vi "svfa_Check for Zoom Settings Change (1 Ch).vi"(6 "zoom settings":T2={"frequency range"={"start frequency"=1000.0, "stop frequency"=2000.0}, "window"=1, "number of lines"=400, "% overlap"=0.0} {"% overlap" min=0.0 format="%.2f"; "number of lines" min=2; "window" items=["None ", "Hanning", "Hamming", "Blackman-Harris", "Exact Blackman", "Blackman", "Flat Top", "4 Term B-Harris ", "7 Term B-Harris", "Low Sidelobe"]; "frequency range"."stop frequency" min=0.0 format="%.2f"; "frequency range"."start frequency" min=0.0 format="%.2f"}, 7 "restart averaging (F)":bool, 8 "error in (no error)":errorcluster, 9 "array length":i32, 10 "dt":dbl) -> (0 "error out":errorcluster, 1 "maximum block size":i32, 2 "zoom settings changed":bool, 3 "iterations":i32, 4 "zoom FFT settings":T1={"zoom settings"={"center frequency"=-inf, "zoom"=1, "trim"=1.0}, "FFT settings"={"window"=enum."Hanning", "window size"=-1, "FFT size"=1024, "%overlap"=0.0}} {"FFT settings"."%overlap" min=0.0 max=100.0 format="%.2f"; "zoom settings"."trim" min=1.0 format="%.2f"; "zoom settings"."center frequency" format="%.2f"; "zoom settings"."zoom" min=1})   [LabVIEW 2017]
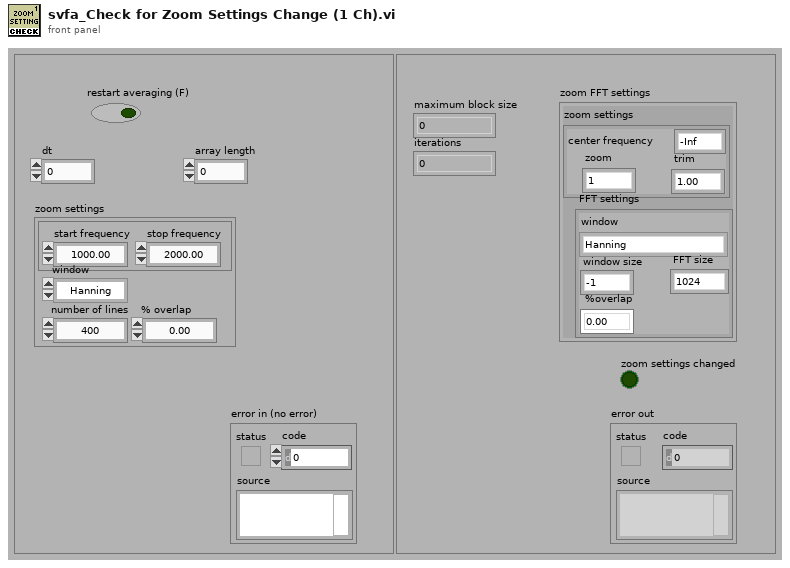
[diagram p1: front panel]
types:
  T1 = cluster{"zoom settings":cluster{"center frequency":dbl, "zoom":i32, "trim":dbl}, "FFT settings":cluster{"window":enum16{"None ", "Hanning", "Hamming", "Blackman-Harris", "Exact Blackman", "Blackman", "Flat Top", "4 Term B-Harris ", "7 Term B-Harris", "Low Sidelobe"}, "window size":i32, "FFT size":i32, "%overlap":dbl}}
  T2 = cluster{"frequency range":cluster{"start frequency":dbl, "stop frequency":dbl}, "window":u16, "number of lines":i32, "% overlap":dbl}
  T3 = cluster{"start frequency":dbl, "stop frequency":dbl}
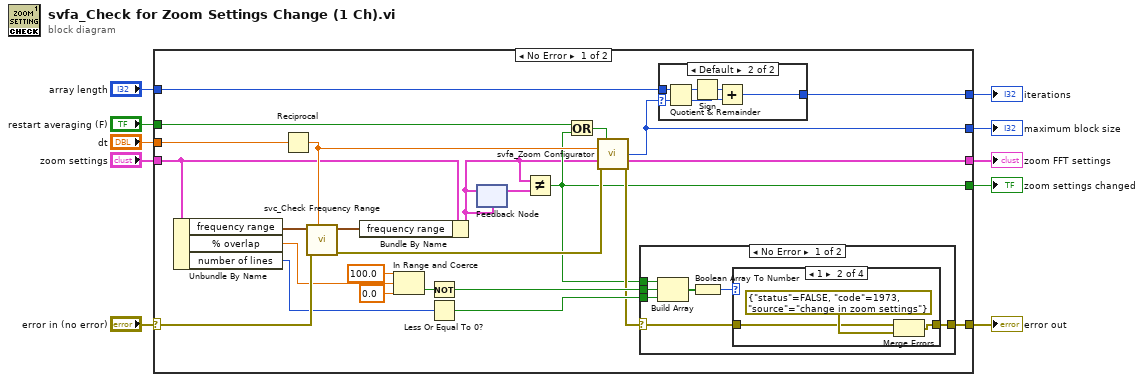
[diagram p0: block diagram]
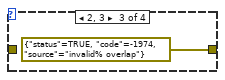
[diagram p4: hidden frame]
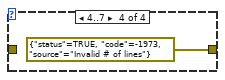
[diagram p5: hidden frame]
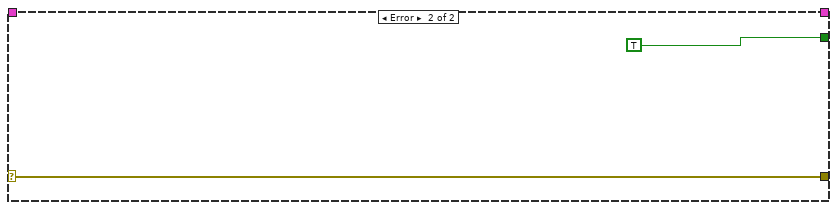
[diagram p7: hidden frame]
diagram:
  n1 = case shown="No Error" "error in (no error)" {
    selector: "error in (no error)" -> [w30 w58]
    tunnel: "zoom settings" -> [w15 _]
    tunnel: [w17 TRUE] -> w9
    tunnel: [w34 w58] -> w7
    tunnel: [w19 _] -> w6
    tunnel: "dt" -> [w28 _]
    tunnel: "array length" -> [w21 _]
    tunnel: [w14 _] -> w3
    tunnel: [w13 _] -> w2
    tunnel: "restart averaging (F)" -> [w20 _]
    frame No Error {
      n2 = Unbundle By Name(w15) -> ("frequency range"=w25:T3, "% overlap"=w26:dbl, "number of lines"=w16:i32)
      n3 = Reciprocal(x=w28) -> (1/x=w22:dbl)
      n4 = call <vilib>:"svc_Check Frequency Range.vi"("fs"=w22, "error in (no error)"=w30, "frequency range in"=w25) -> ("error out"=w24:errorcluster, "frequency range out"=w29:T3)  [unwired: 6 in, 1 out]
      n5 = Bundle By Name(cluster=w15, "frequency range"=w29) -> (w12:T2)
      n6 = In Range and Coerce(upper limit=100.0, x=w26, lower limit=0.0) -> (In Range?=w32:bool)  [unwired: 1 out]
      n7 = Not(x=w32) -> (.not. x?=w27:bool)
      n8 = Less Or Equal To 0?(x=w16) -> (x <= 0?=w33:bool)
      n9 = feedback-in #1(w12) -> ()
      n10 = feedback #1(w12) -> (w11:T2)
      n11 = Not Equal?(x=w12, y=w11) -> (x != y?=w17:bool)
      n12 = Or(x=w20, y=w17) -> (x .or. y?=w18:bool)
      n13 = call <vilib>:"svfa_Zoom Configurator.vi"("restart averaging (F)"=w18, "fs"=w22, "zoom settings"=w12, "error in (no error)"=w24) -> ("Max Block Size"=w13:i32, "zoom FFT settings"=w19:T1, "error out"=w23:errorcluster)  [unwired: 8 in, 1 out]
      n14 = case shown="No Error" w23 {
        selector: w23 -> [w48 w56]
        tunnel: [w43 w56] -> w34
        tunnel: w33 -> [w49 _]
        tunnel: w27 -> [w47 _]
        tunnel: w17 -> [w46 _]
        frame No Error {
          n15 = Build Array(w46, w47, w49) -> (w45:bool[])
          n16 = Boolean Array To Number(Boolean array=w45) -> (number=w44:u32)
          n17 = case shown="1" w44 {
            tunnel: [w50 w53 errorcluster {"status"=TRUE, "code"=-1974, "source"="invalid% overlap"} ("error IO") errorcluster {"status"=TRUE, "code"=-1973, "source"="Invalid # of lines"} ("error IO")] -> w43
            tunnel: w48 -> [w50 w51 _ _]
            frame 0, Default {
            }
            frame 1 {
              n18 = Merge Errors(w51, errorcluster {"status"=FALSE, "code"=1973, "source"="change in zoom settings"} ("error IO")) -> (w53:errorcluster)
            }
            frame 2, 3 {
            }
            frame 4..7 {
            }
          }
        }
        frame Error {
        }
      }
      n19 = case shown="Default" w13 {
        selector: w13 -> [w36 w41]
        tunnel: w21 -> [_ w42]
        tunnel: [w36 w37] -> w14
        frame 0 {
        }
        frame Default {
          n20 = Quotient & Remainder(x=w42, y=w41) -> (x-y*floor(x/y)=w40:i32, floor(x/y)=w38:i32)
          n21 = Sign(1:w40) -> (0:w39:i32)
          n22 = Add(x=w39, y=w38) -> (x+y=w37:i32)
        }
      }
    }
    frame Error {
    }
  }
  "error out" <- w7
  "zoom settings changed" <- w9
  "zoom FFT settings" <- w6
  "maximum block size" <- w2
  "iterations" <- w3
